vi "Cycle.vi"(8 "error in (no error)":errorcluster, 11 "MatlabExperiment In":refnum<class "MatlabExperiment.lvclass">) -> (0 "error out":errorcluster, 3 "MatlabExperiment Out":refnum<class "MatlabExperiment.lvclass">)   [LabVIEW 2012, in "AcquisitionCoreLibrary.lvlib" / "MatlabExperiment.lvclass"]
uses:
  MatlabExperiment.lvclass
  TrialBasedExperimentObject/TrialBasedExperiment.lvclass
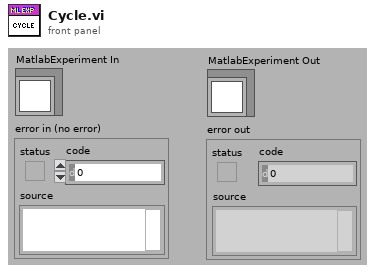
[diagram p1: front panel]
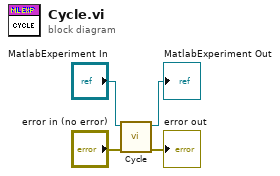
[diagram p0: block diagram]
diagram:
  n1 = call-parent "Cycle.vi"("error in (no error)"="error in (no error)", "TrialBasedExperiment In"="MatlabExperiment In") -> ("error out"=→"error out":errorcluster, "TrialBasedExperiment Out"=→"MatlabExperiment Out":refnum<class "MatlabExperiment.lvclass">)  [unwired: 8 in]
